vi "FRCts20_Backend_Event_DELETE.vi"(8 "error in (no error)":errorcluster, 11 "Name":string) -> (0 "error out":errorcluster, 1 "Time (ms)":u32, 2 "Status":string, 3 "Event Out":T1, 5 "Success":bool)   [LabVIEW 2014, in "FRCts20_Backend_TestCode.lvlib"]
uses:
  FRCts20_Backend_TestCode.lvlib
  FRCts20_Backend_API/FRCts20_Backend_API_Event.ctl
  FRCts20_Backend_API/FRCts20_Backend_API.lvlib
  FRCts20_Backend_API/FRCts20_Backend_API_Command_Event.ctl
  FRCts20_Backend_API/FRCts20_Backend_API_Event.vi
  FRCts20_Backend_API/FRCts20_Backend_API_SW.ctl
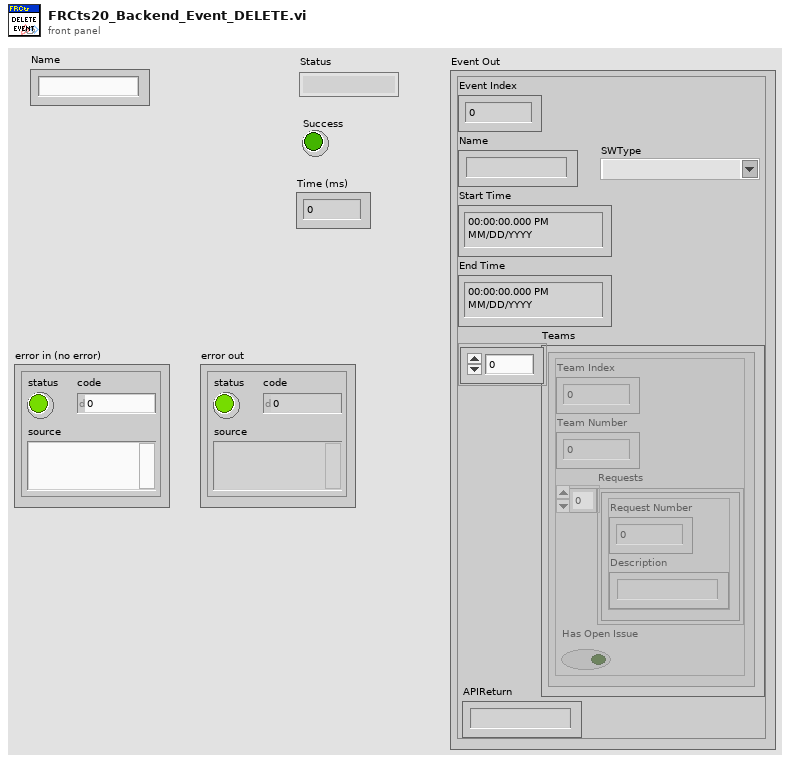
[diagram p1: front panel]
types:
  T1 = typedef "FRCts20_Backend_API.lvlib/FRCts20_Backend_API_Event.ctl" = cluster{"Event Index":u32, "Name":string, "Start Time":timestamp, "End Time":timestamp, "Teams":cluster{"Team Index":u32, "Team Number":u32, "Requests":cluster{"Request Number":u32, "Description":string}[], "Has Open Issue":bool}[], "SWType":T2, "APIReturn":string}
  T2 = typedef "FRCts20_Backend_API.lvlib/FRCts20_Backend_API_SW.ctl" = string
  T3 = typedef "FRCts20_Backend_API.lvlib/FRCts20_Backend_API_Command_Event.ctl" = string
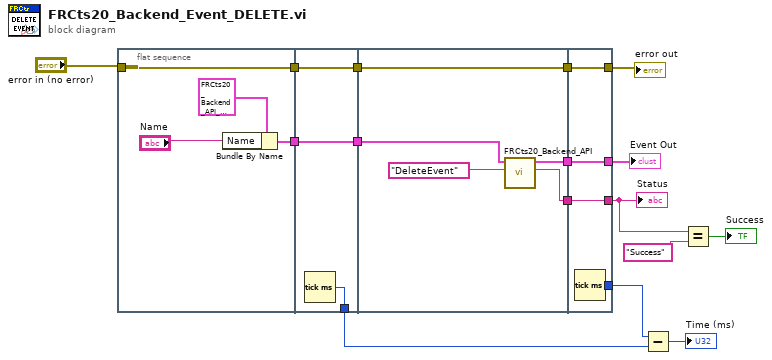
[diagram p0: block diagram]
diagram:
  n1 = flat-sequence {
    tunnel: "error in (no error)" -> [w20]
    tunnel: [w20] -> w16
    tunnel: [w19] -> w15
    tunnel: [w23] -> w3
    tunnel: [w22] -> w14
    tunnel: w16 -> [w22]
    tunnel: [w21] -> w13
    tunnel: w15 -> [w21]
    tunnel: [w28] -> w12
    tunnel: w14 -> [w28]
    tunnel: w13 -> [w26]
    tunnel: [w25] -> w11
    tunnel: [w24] -> w10
    tunnel: [w32] -> w4
    tunnel: [w31] -> w6
    tunnel: w12 -> [w31]
    tunnel: [w30] -> w2
    tunnel: w11 -> [w30]
    tunnel: [w29] -> w1
    tunnel: w10 -> [w29]
    frame #0 {
      n2 = Bundle By Name(cluster=T1 {"Event Index"=0, "Name"="", "Start Time"=timestamp(0 s since 1904-01-01), "End Time"=timestamp(0 s since 1904-01-01), "Teams"=[], "SWType"="", "APIReturn"=""} ("Event In"), "Name"="Name") -> (w19:T1)
    }
    frame #1 {
      n3 = Tick Count (ms)() -> (millisecond timer value=w23:u32)
    }
    frame #2 {
      n4 = call-poly "FRCts20_Backend_API.vi"("Command"=T3 "DeleteEvent", "Event In"=w26) -> ("Status"=w24:string, "Event Out"=w25:T1)  [unwired: 7 in, 1 out]
    }
    frame #3 {
      n5 = Tick Count (ms)() -> (millisecond timer value=w32:u32)
    }
  }
  n6 = Subtract(x=w4, y=w3) -> (x-y=→"Time (ms)":u32)
  n7 = Equal?(x=w1, y="Success") -> (x = y?=→"Success":bool)
  "Event Out" <- w2
  "Status" <- w1
  "error out" <- w6
